vi "Configure.vi"(8 "error in (no error)":errorcluster, 10 "Msg in":T1, 11 "FakePressureController in":refnum<class "DaqPad_NI6009.lvclass">) -> (0 "error out":errorcluster, 1 "new command":string, 2 "Msg out":T1, 3 "FakePressureController out":refnum<class "DaqPad_NI6009.lvclass">)   [LabVIEW 2011, in "DaqPad_NI6009.lvclass"]
uses:
  DaqPad_NI6009.lvclass
  DriverMsg.ctl
  DaqPad_NI6009.lvclass/DaqPad_NI6009.ctl
  OnOffTypeDef.ctl
  BaseDriver/BaseDriver.lvclass
  DAQmx Fill In Error Info.vi
  C:/Program Files/National Instruments/LabVIEW 2011/resource/objmgr/daqmx.rc
panel:
  out "number":dbl
  out "NumChans":u32
  out "Channels":refnum<k21>[](array[refnum])
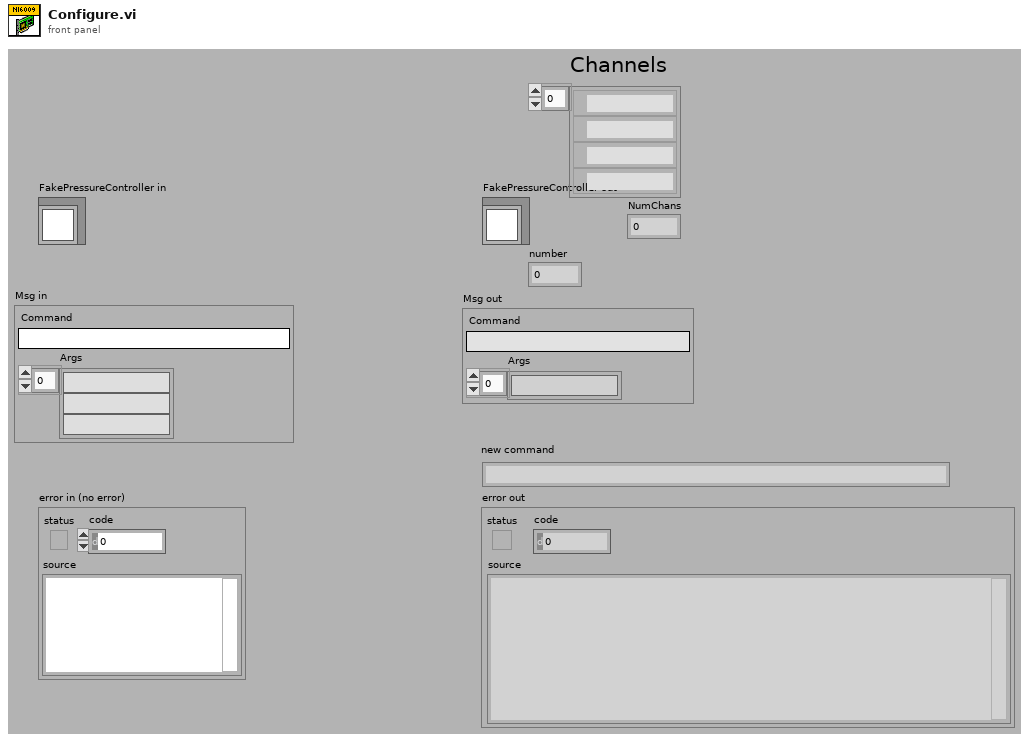
[diagram p1: front panel]
types:
  T1 = typedef "DriverMsg.ctl" = cluster{"Command":string, "Args":string[]}
  T2 = typedef "OnOffTypeDef.ctl" = enum16{"off", "on"}
  T3 = typedef "numericVariable_TypeDef.ctl" = cluster{"Value":dbl, "Min":dbl, "Max":dbl, "StepSize":dbl, "Tolerance":dbl, "valueactual":dbl}
  T4 = cluster{"Channel 0":T3, "Channel 1":T3, "Channel 2":T3, "Channel 3":T3, "Channel 4":T3, "Channel 5":T3, "Channel 6":T3, "Channel 7":T3}
  T5 = cluster{"Channel 0":T2, "Channel 1":T2, "Channel 2":T2, "Channel 3":T2}
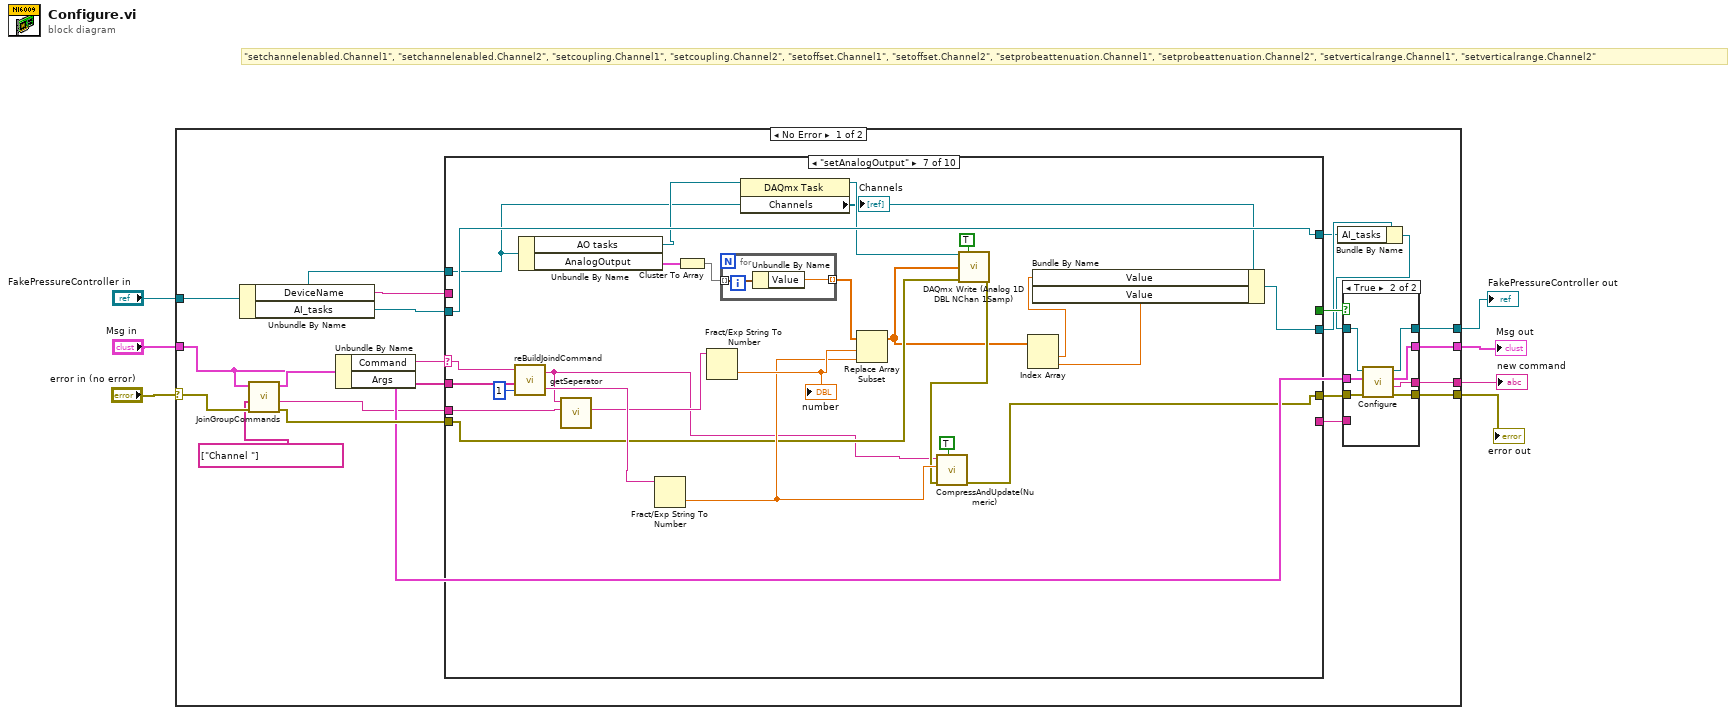
[diagram p0: block diagram]
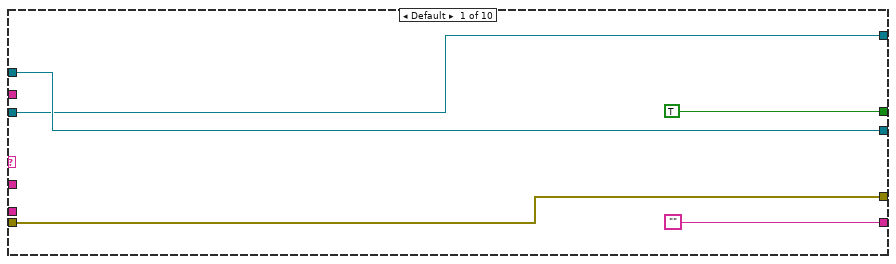
[diagram p3: hidden frame]
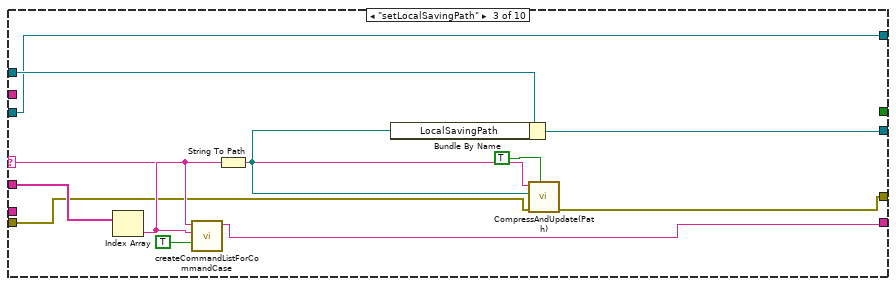
[diagram p5: hidden frame]
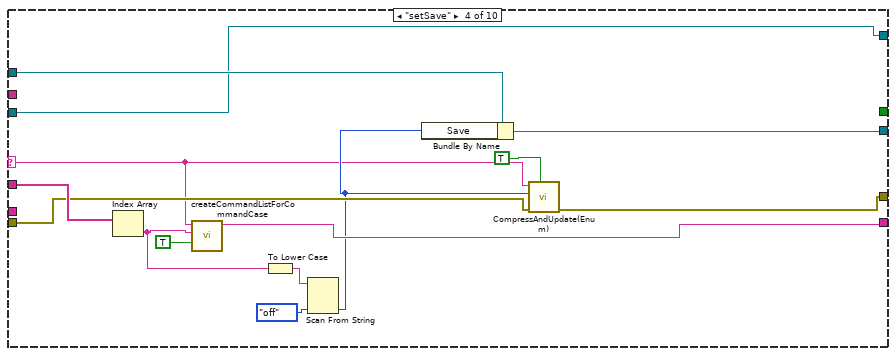
[diagram p6: hidden frame]
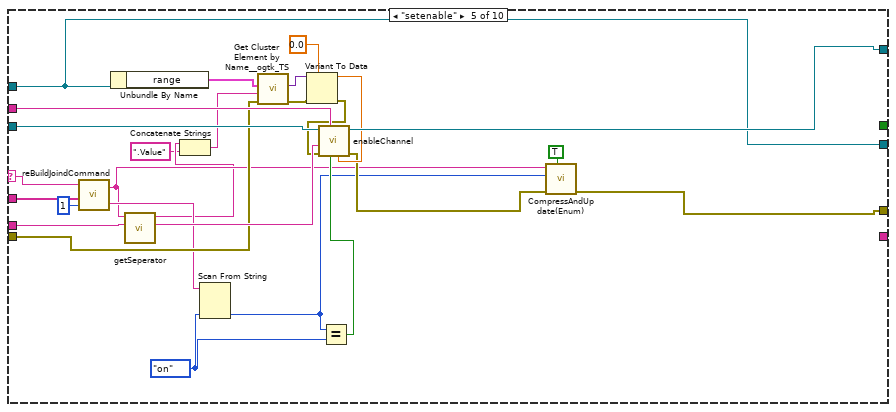
[diagram p7: hidden frame]
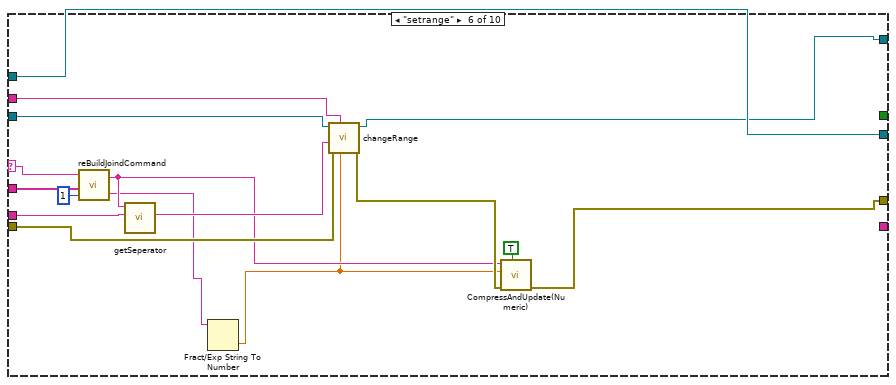
[diagram p8: hidden frame]
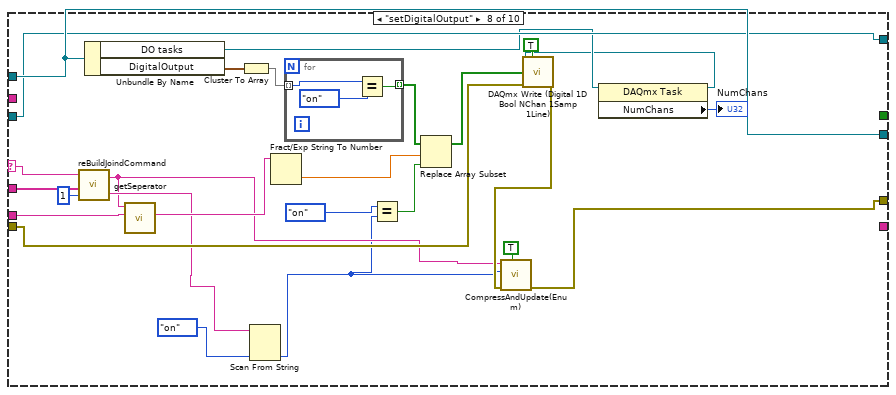
[diagram p9: hidden frame]
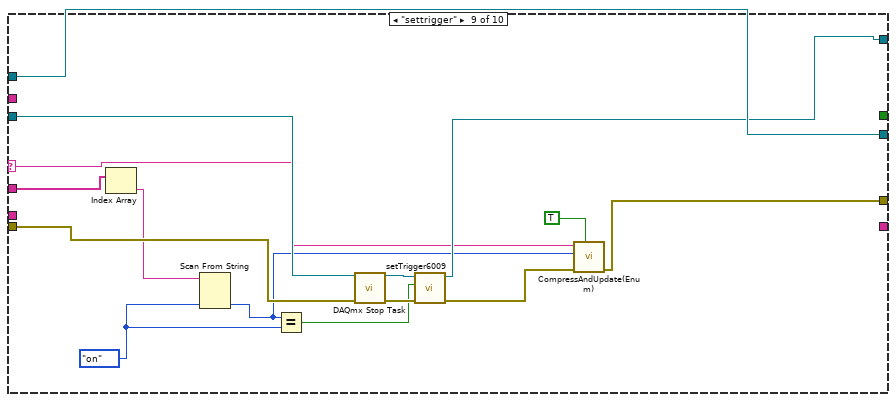
[diagram p10: hidden frame]
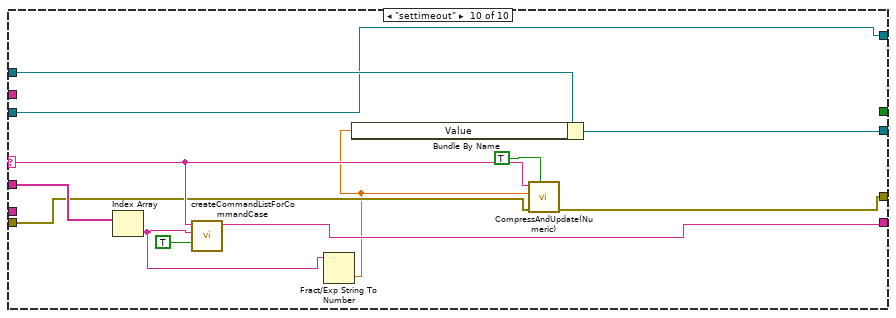
[diagram p11: hidden frame]
diagram:
  # "\"setchannelenabled.Channel1\", \"setchannelenabled.Channel2\", \"setcoupling.Channel1\", \"setcoupling.Channel2\", \"setoffset.Channel1\", \"setoffset.Channel2\", \"setprobeattenuation.Channel1\", \"setprobeattenuation.Channel2\", \"setverticalrange.Channel1\", \"setverticalrange.Channel2\""
  n1 = case shown="No Error" "error in (no error)" {
    selector: "error in (no error)" -> [w17 w203]
    tunnel: "FakePressureController in" -> [w20 w201]
    tunnel: [w28 w201] -> w4
    tunnel: [w26 w203] -> w1
    tunnel: "Msg in" -> [w14 w202]
    tunnel: [w24 w202] -> w3
    tunnel: [w22 _] -> w2
    frame No Error {
      n2 = Unbundle By Name(w20) -> ("DeviceName"=w8:string, "AI_tasks"=w19:refnum<k21>)
      n3 = call "JoinGroupCommands.vi"("error in (no error)"=w17, "Seperator"=string[] ["Channel "], "Msg in"=w14) -> ("error out"=w16:errorcluster, "Seperator out"=w13:string, "Msg out"=w15:T1)  [unwired: 6 in]
      n4 = Unbundle By Name(w15) -> ("Command"=w21:string, "Args"=w18:string[])
      n5 = case shown="\"setAnalogOutput\"" w21 {
        selector: w21 -> [_ _ w54 w61 w100 w116 w142 w170 w174 w196]
        tunnel: w16 -> [w43 w46 w51 w68 w90 w108 w128 w157 w183 w194]
        tunnel: w18 -> [_ _ w57 w71 w99 w115 w141 w169 w182 w198]
        tunnel: w20 -> [w44 w47 w59 w73 w85 w113 w121 w164 w188 w200]
        tunnel: [w44 w47 w49 w66 w85 w113 w117 w164 w188 w192] -> w11
        tunnel: ["" ("Complete") _ w55 w70 _ _ _ _ _ w197] -> w23
        tunnel: [w43 w46 w50 w67 w79 w105 w138 w166 w176 w193] -> w27
        tunnel: [TRUE _ _ _ _ _ _ _ _ _] -> w25
        tunnel: w19 -> [w40 w45 w48 w60 w97 w112 w126 w148 w185 w189]
        tunnel: w13 -> [_ _ _ _ w98 w114 w140 w168 _ _]
        tunnel: [w40 w45 w48 w60 w96 w111 w126 w148 w184 w189] -> w9
        tunnel: w8 -> [_ _ _ _ w94 w110 _ _ _ _]
        frame Default {
        }
        frame "Abort" {
        }
        frame "setLocalSavingPath" {
          n6 = Index Array(array=w57) -> (element=w56:string)  [unwired: 1 in]
          n7 = call "createCommandListForCommandCase.vi"("immediate Check (only once)"=TRUE, "setvalue"=w56, "command"=w54) -> ("new commands"=w55:string)  [unwired: 8 in]
          n8 = String To Path(string=w56) -> (path=w53:path)
          n9 = Bundle By Name(cluster=w59, "LocalSavingPath"=w53) -> (w49:refnum<class "DaqPad_NI6009.lvclass">)
          n10 = call "CompressAndUpdate(Path).vi"("force CVT update (false)"=TRUE, "error in"=w51, "Path"=w53, "command or variable name"=w54) -> ("error out"=w50:errorcluster)  [unwired: 7 in]
        }
        frame "setSave" {
          n11 = Index Array(array=w71) -> (element=w63:string)  [unwired: 1 in]
          n12 = call "createCommandListForCommandCase.vi"("immediate Check (only once)"=TRUE, "setvalue"=w63, "command"=w61) -> ("new commands"=w70:string)  [unwired: 8 in]
          n13 = To Lower Case(string=w63) -> (all lower case string=w65:string)
          n14 = Scan From String(input string=w65, default 1=OnOffTypeDef."off" ("Settings.Trigger")) -> (output 1=w62:T2)  [unwired: 3 in, 3 out]
          n15 = Bundle By Name(cluster=w73, "Save"=w62) -> (w66:refnum<class "DaqPad_NI6009.lvclass">)
          n16 = call "CompressAndUpdate(Enum).vi"("force CVT update (false)"=TRUE, "error in"=w68, "enum variant"=w62, "command or variable name"=w61) -> ("error out"=w67:errorcluster)  [unwired: 7 in]
        }
        frame "setenable" {
          w93 = OnOffTypeDef."on" ("Channel 0")
          n17 = call "reBuildJoindCommand.vi"("number of group elements (0)"=1, "Args"=w99, "Command 2"=w100) -> ("Arg"=w84:string, "Command"=w81:string)
          n18 = Unbundle By Name(w85) -> ("range"=w91:T4)
          n19 = call "getSeperator.vi"("Channel Seperator (\"\")"=w98, "Command"=w81) -> ("Channel"=w95:string, "Seperator (e.g. \"Channel1\")"=w77:string)  [unwired: 8 in]
          n20 = Concatenate Strings(w77, ".Value" ("string")) -> (w75:string)
          n21 = Scan From String(input string=w84, default 1=w93) -> (output 1=w82:T2)  [unwired: 3 in, 3 out]
          n22 = call "Get Cluster Element by Name__ogtk_TS.vi"("error in (no error)"=w90, "Element Name"=w75, "Cluster"=w91) -> ("error out"=w87:errorcluster, "VElement"=w89:variant)  [unwired: 6 in, 1 out]
          n23 = Variant To Data(error in=w87, type=0.0, Variant=w89) -> (data=w88:dbl, error out=w86:errorcluster)
          n24 = Equal?(x=w82, y=w93) -> (x = y?=w92:bool)
          n25 = call "enableChannel.vi"("range"=w88, "Enable"=w92, "Device Name"=w94, "error in (no error)"=w86, "Channel (0.1.2.3)"=w95, "Refnum in"=w97) -> ("error out"=w83:errorcluster, "Refnum out"=w96:refnum<k21>)  [unwired: 4 in]
          n26 = call "CompressAndUpdate(Enum).vi"("force CVT update (false)"=TRUE, "error in"=w83, "enum variant"=w82, "command or variable name"=w81) -> ("error out"=w79:errorcluster)  [unwired: 7 in]
        }
        frame "setrange" {
          n27 = call "reBuildJoindCommand.vi"("number of group elements (0)"=1, "Args"=w115, "Command 2"=w116) -> ("Arg"=w102:string, "Command"=w104:string)
          n28 = call "getSeperator.vi"("Channel Seperator (\"\")"=w114, "Command"=w104) -> ("Channel"=w109:string)  [unwired: 8 in, 1 out]
          n29 = Fract/Exp String To Number(string=w102) -> (number=w101:dbl)  [unwired: 3 in, 1 out]
          n30 = call "changeRange.vi"("range (V)"=w101, "Device Name"=w110, "error in (no error)"=w108, "Channel (0.1.2.3)"=w109, "Refnum in"=w112) -> ("error out"=w106:errorcluster, "Refnum out"=w111:refnum<k21>)  [unwired: 4 in, 1 out]
          n31 = call "CompressAndUpdate(Numeric).vi"("force CVT update (false)"=TRUE, "error in"=w106, "Numeric"=w101, "command or variable name"=w104) -> ("error out"=w105:errorcluster)  [unwired: 7 in]
        }
        frame "setAnalogOutput" {
          n32 = call "reBuildJoindCommand.vi"("number of group elements (0)"=1, "Args"=w141, "Command 2"=w142) -> ("Arg"=w135:string, "Command"=w122:string)
          n33 = Unbundle By Name(w121) -> ("AO tasks"=w125:refnum<k21>, "AnalogOutput"=w134:cluster{"Channel 0":T3, "Channel 1":T3})
          n34 = call "getSeperator.vi"("Channel Seperator (\"\")"=w140, "Command"=w122) -> ("Channel"=w131:string)  [unwired: 8 in, 1 out]
          n35 = Fract/Exp String To Number(string=w135) -> (number=w129:dbl)  [unwired: 3 in, 1 out]
          n36 = Cluster To Array(cluster=w134) -> (array=w133:T3[])
          n37 = Fract/Exp String To Number(string=w131) -> (number=w130:dbl)  [unwired: 3 in, 1 out]
          "number" <- w130
          n38 = for {
            tunnel: w133 -> [w144] mode=indexing
            tunnel: [w143] -> w132 mode=indexing
            n39 = Unbundle By Name(w144) -> ("Value"=w143:dbl)
          }
          n40 = property class="DAQmx Task"(reference=w125) -> (reference out=w124:refnum<k21>, "Channels"=→"Channels":refnum<k21>[])  [unwired: 1 in, 1 out]
          n41 = Replace Array Subset(array=w132, new element=w129, index=w130) -> (w120:dbl[])
          n42 = call "DAQmx Write (Analog 1D DBL NChan 1Samp).vi"("task/channels in"=w124, "auto start"=TRUE, "data"=w120, "error in"=w128) -> ("error out"=w127:errorcluster)  [unwired: 9 in, 2 out]
          n43 = call "CompressAndUpdate(Numeric).vi"("force CVT update (false)"=TRUE, "error in"=w127, "Numeric"=w129, "command or variable name"=w122) -> ("error out"=w138:errorcluster)  [unwired: 7 in]
          n44 = Index Array(array=w120) -> (element #1=w119:dbl, element #2=w118:dbl)  [unwired: 2 in]
          n45 = Bundle By Name(cluster=w121, "Value"=w119, "Value"=w118) -> (w117:refnum<class "DaqPad_NI6009.lvclass">)
        }
        frame "setDigitalOutput" {
          n46 = call "reBuildJoindCommand.vi"("number of group elements (0)"=1, "Args"=w169, "Command 2"=w170) -> ("Arg"=w155:string, "Command"=w153:string)
          n47 = Unbundle By Name(w164) -> ("DO tasks"=w147:refnum<k21>, "DigitalOutput"=w162:T5)
          n48 = call "getSeperator.vi"("Channel Seperator (\"\")"=w168, "Command"=w153) -> ("Channel"=w159:string)  [unwired: 8 in, 1 out]
          n49 = Cluster To Array(cluster=w162) -> (array=w161:T2[])
          n50 = Scan From String(input string=w155, default 1=OnOffTypeDef."on" ("y")) -> (output 1=w151:T2)  [unwired: 3 in, 3 out]
          n51 = Fract/Exp String To Number(string=w159) -> (number=w158:dbl)  [unwired: 3 in, 1 out]
          n52 = for {
            tunnel: w161 -> [w173] mode=indexing
            tunnel: [w171] -> w160 mode=indexing
            n53 = Equal?(x=w173, y=OnOffTypeDef."on") -> (x = y?=w171:bool)
          }
          n54 = Equal?(x=OnOffTypeDef."on" ("y"), y=w151) -> (x = y?=w150:bool)
          n55 = Replace Array Subset(array=w160, new element=w150, index=w158) -> (w149:bool[])
          n56 = property class="DAQmx Task"(reference=w147) -> (reference out=w146:refnum<k21>, "NumChans"=→"NumChans":u32)  [unwired: 1 in, 1 out]
          n57 = call "DAQmx Write (Digital 1D Bool NChan 1Samp 1Line).vi"("task/channels in"=w146, "auto start"=TRUE, "data"=w149, "error in"=w157) -> ("error out"=w156:errorcluster)  [unwired: 9 in, 2 out]
          n58 = call "CompressAndUpdate(Enum).vi"("force CVT update (false)"=TRUE, "error in"=w156, "enum variant"=w151, "command or variable name"=w153) -> ("error out"=w166:errorcluster)  [unwired: 7 in]
        }
        frame "settrigger" {
          w181 = OnOffTypeDef."on" ("Channel 0")
          n59 = Index Array(array=w182) -> (element=w179:string)  [unwired: 1 in]
          n60 = Scan From String(input string=w179, default 1=w181) -> (output 1=w178:T2)  [unwired: 3 in, 3 out]
          n61 = Equal?(x=w178, y=w181) -> (x = y?=w180:bool)
          n62 = call "DAQmx Stop Task.vi"("task/channels in"=w185, "error in"=w183) -> ("task out"=w186:refnum<k21>, "error out"=w187:errorcluster)  [unwired: 12 in]
          n63 = call "setTrigger6009.vi"("error in (no error)"=w187, "Trigger"=w180, "Refnum in"=w186) -> ("error out"=w177:errorcluster, "Refnum out"=w184:refnum<k21>)  [unwired: 6 in, 1 out]
          n64 = call "CompressAndUpdate(Enum).vi"("force CVT update (false)"=TRUE, "error in"=w177, "enum variant"=w178, "command or variable name"=w174) -> ("error out"=w176:errorcluster)  [unwired: 7 in]
        }
        frame "settimeout" {
          n65 = Index Array(array=w198) -> (element=w191:string)  [unwired: 1 in]
          n66 = call "createCommandListForCommandCase.vi"("immediate Check (only once)"=TRUE, "setvalue"=w191, "command"=w196) -> ("new commands"=w197:string)  [unwired: 8 in]
          n67 = Fract/Exp String To Number(string=w191) -> (number=w190:dbl)  [unwired: 3 in, 1 out]
          n68 = Bundle By Name(cluster=w200, "Value"=w190) -> (w192:refnum<class "DaqPad_NI6009.lvclass">)
          n69 = call "CompressAndUpdate(Numeric).vi"("force CVT update (false)"=TRUE, "error in"=w194, "Numeric"=w190, "command or variable name"=w196) -> ("error out"=w193:errorcluster)  [unwired: 7 in]
        }
      }
      n70 = Bundle By Name(cluster=w11, "AI_tasks"=w9) -> (w10:refnum<class "DaqPad_NI6009.lvclass">)
      n71 = case shown="True" w25 {
        tunnel: w10 -> [w30 w39]
        tunnel: [w30 w38] -> w28
        tunnel: [w31 w37] -> w22
        tunnel: w27 -> [w29 w36]
        tunnel: [w29 w35] -> w26
        tunnel: w14 -> [w32 w34]
        tunnel: [w32 w33] -> w24
        tunnel: w23 -> [w31 _]
        frame False {
        }
        frame True {
          n72 = call-parent "Configure.vi"("error in (no error)"=w36, "Msg in"=w34, "BaseDriver in"=w39) -> ("error out"=w35:errorcluster, "new command"=w37:string, "Msg out"=w33:T1, "BaseDriver out"=w38:refnum<class "DaqPad_NI6009.lvclass">)  [unwired: 5 in]
        }
      }
    }
    frame Error {
    }
  }
  "error out" <- w1
  "FakePressureController out" <- w4
  "new command" <- w2
  "Msg out" <- w3
